vi "Create Master Instance.vi"   [LabVIEW 2020, in "Modbus Master.lvclass"]
doc: "Creates a serial or TCP Modbus master instance. You must manually select the polymorphic instance to use."
uses:
  <vilib>/Modbus/master/Modbus Master.lvclass
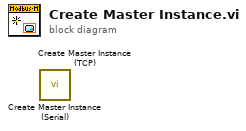
[diagram p0: block diagram]
diagram:
  n1 = call <vilib>:"Create Master Instance (Serial).vi"() -> ()  [unwired: 10 in, 2 out]
  n2 = call <vilib>:"Create Master Instance (TCP).vi"() -> ()  [unwired: 10 in, 2 out]
